vi "Is Concrete Class.vi"(0 "SG 8GHz Path Group in":refnum<class "SG 8GHz Path Group.lvclass">, 11 "error in":errorcluster) -> (4 "SG 8GHz Path Group out":refnum<class "SG 8GHz Path Group.lvclass">, 6 "Is Concrete Class?":bool, 15 "error out":errorcluster)   [LabVIEW 2023, in "RFFixtureCharact.PXI.lvlib" / "SG 8GHz Path Group.lvclass"]
uses:
  SG 8GHz Path Group.lvclass
  SG 8GHz Path Group.lvclass/SG 8GHz Path Group.ctl
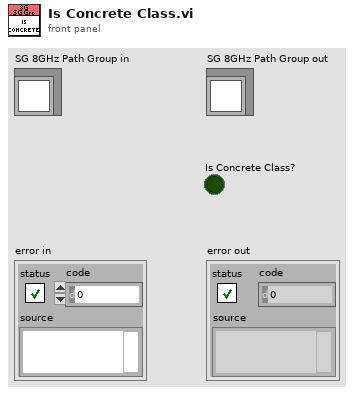
[diagram p1: front panel]
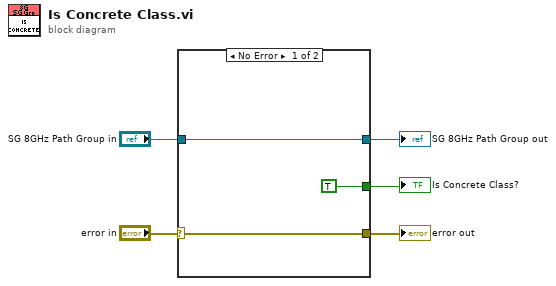
[diagram p0: block diagram]
diagram:
  n1 = case shown="No Error" "error in" {
    selector: "error in" -> [w7 w10]
    tunnel: [TRUE ("Is Concrete Class?") _] -> w3
    tunnel: [w7 w10] -> w4
    tunnel: "SG 8GHz Path Group in" -> [w6 w9]
    tunnel: [w6 w9] -> w2
    frame No Error {
    }
    frame Error {
    }
  }
  "error out" <- w4
  "SG 8GHz Path Group out" <- w2
  "Is Concrete Class?" <- w3
